vi "clear_multi_turn.vi"() -> ()   [LabVIEW 2016]
uses:
  dxl_x86_c.lvlib/dxl_x86_c.lvlib
panel:
  out "?":string
  in  "?":bool
  out "value : PRO (knob)\npresent position 2":i32(knob)
  out "value : PRO (knob)\npresent position":i32(knob) scale=150000.0..-150000.0
  in  "?":bool
  out "?":string
  in  "MAX_POSITION_VALUE":u32=1048575
  out "EXT_POSITION_\nCONTROL_MODE":dbl=4.0
  out "ADDR_\nOPERATING_MODE":u16
  in  "?":bool
  out "dynamixel_comm_result":string
  out "dynamixel_error":string
  in  "device_name":string="COM1"
  in  "ADDR_\nPRESENT_POSITION":u16=611
  in  "ADDR_\nGOAL_POSITION":u16=596
  in  "ADDR_\nTORQUE_ENABLE":u16=562
  out "protocol_version":dbl=2.0
  in  "?":bool
  out "port_num":i32
  in  "dynamixel_id":u8=1
  in  "baud_rate":i32=57600
  # "/*******************************************************************************\n* Copyright (c) 2016, ROBOTIS CO., LTD.\n* All rights reserved.\n*\n* Redistribution and use in source and binary forms, with or without\n* modification, are permitted provided that the following conditions are met:\n*\n* * Redistributions of source code must retain the above copyright notice, this\n*   list of conditions and the following disclaimer.\n*\n* * Redistributions in binary form must reproduce the above copyright notice,\n*   this list of conditions and the following disclaimer in the documentation\n*   and/or other materials provided with the distribution.\n*\n* * Neither the name of ROBOTIS nor the names of its\n*   contributors may be used to endorse or promote products derived from\n*   this software without specific prior written permission.\n*\n* THIS SOFTWARE IS PROVIDED BY THE COPYRIGHT HOLDERS AND CONTRIBUTORS \"AS IS\"\n* AND ANY EXPRESS OR IMPLIED WARRANTIES, INCLUDING, BUT NOT LIMITED TO, THE\n* IMPLIED WARRANTIES OF MERCHANTABILITY AND FITNESS FOR A PARTICULAR PURPOSE ARE\n* DISCLAIMED. IN NO EVENT SHALL THE COPYRIGHT HOLDER OR CONTRIBUTORS BE LIABLE\n* FOR ANY DIRECT, INDIRECT, INCIDENTAL, SPECIAL, EXEMPLARY, OR CONSEQUENTIAL\n* DAMAGES (INCLUDING, BUT NOT LIMITED TO, PROCUREMENT OF SUBSTITUTE GOODS OR\n* SERVICES; LOSS OF USE, DATA, OR PROFITS; OR BUSINESS INTERRUPTION) HOWEVER\n* CAUSED AND ON ANY THEORY OF LIABILITY, WHETHER IN CONTRACT, STRICT LIABILITY,\n* OR TORT (INCLUDING NEGLIGENCE OR OTHERWISE) ARISING IN ANY WAY OUT OF THE USE\n* OF THIS SOFTWARE, EVEN IF ADVISED OF THE POSSIBILITY OF SUCH DAMAGE.\n*******************************************************************************/\n\n/* Author: Ki Jong Gil (Gilbert) */"
  # "Available Dynamixel model on this example : All models using Protocol 2.0\nThis example is designed for using a Dynamixel X Series, and an USB2DYNAMIXEL.\nTo use another Dynamixel model, see their details in E-Manual(support.robotis.com) \nBe sure that Dynamixel X properties are already set as %% ID : 1 / Baudnum : 1 (Baudrate : 57600)\n\n1. Run example by click above \"Run\" button (below \"Edit\" menu).\n2. Click \"Start\" then you may see the Dynamixel and \"knob\" rotating\n3. When you want to clear turn, press \"Clear\" button.\n4. To contiue the turn, press \"Run\" button.\n3. To finish the example, press \"Stop\", \"Run\" and \"terminate\" button."
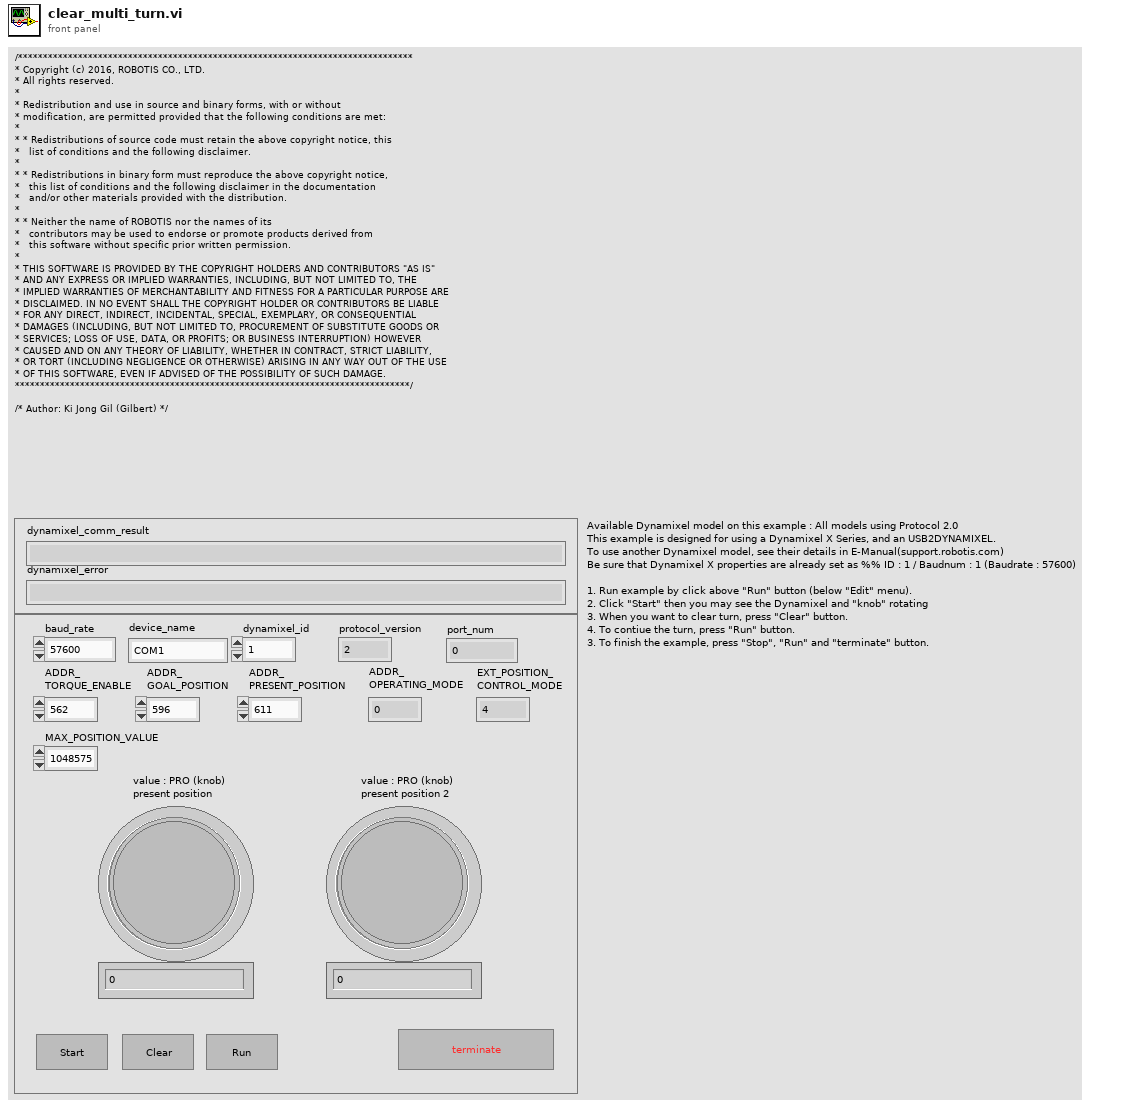
[diagram p1: front panel]
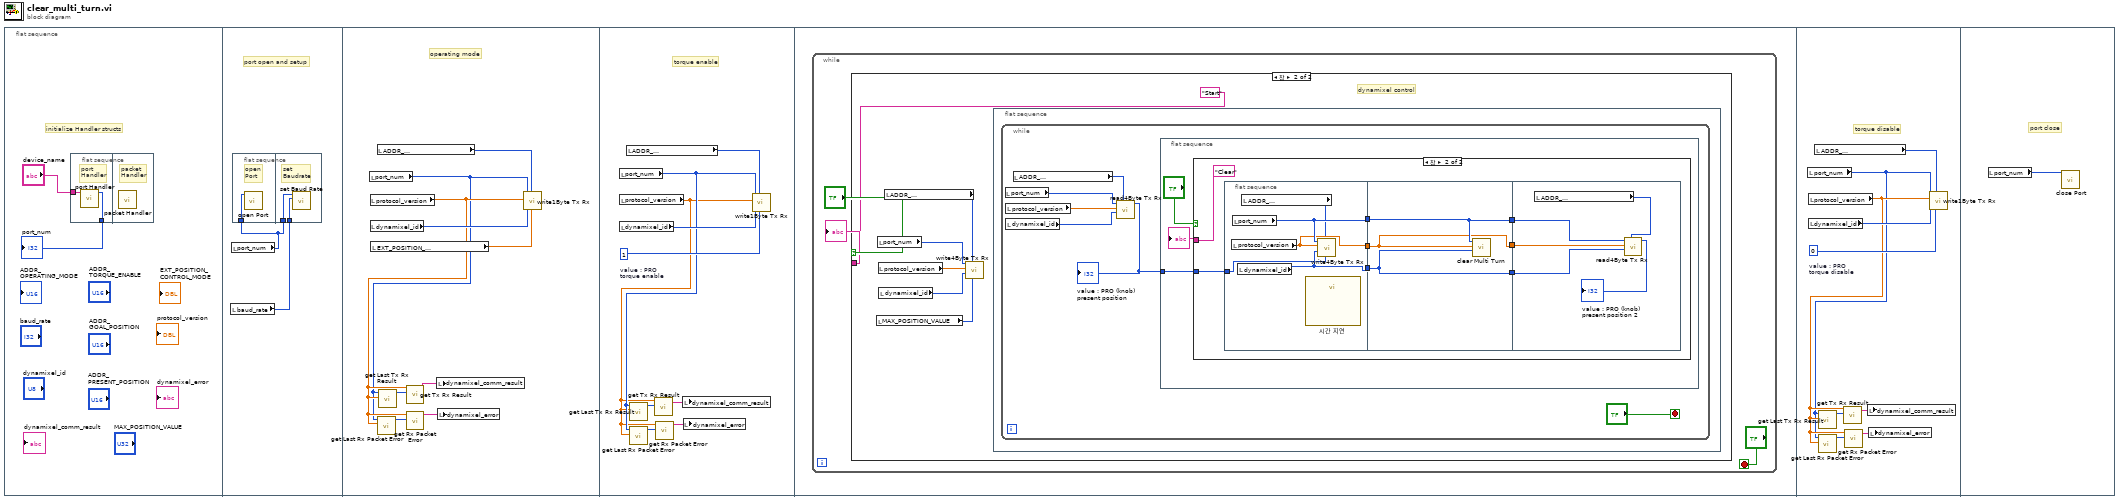
[diagram p0: block diagram]
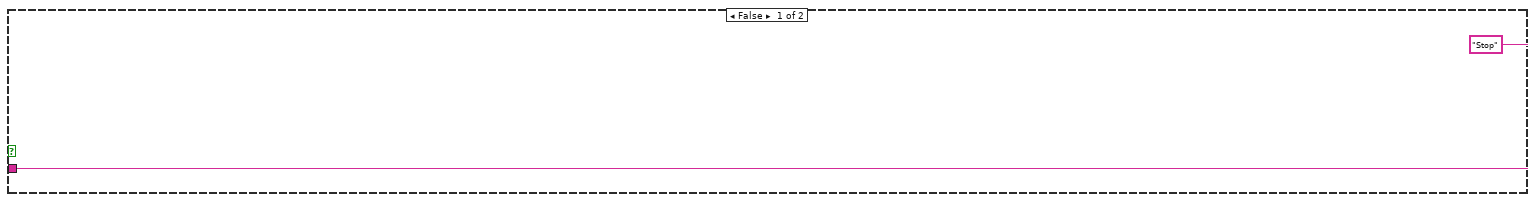
[diagram p2: hidden frame]
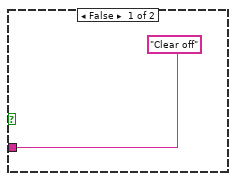
[diagram p3: hidden frame]
diagram:
  n1 = flat-sequence {
    frame #0 {
      # "initialize Handler structs"
      n2 = flat-sequence {
        tunnel: [w4] -> w2
        tunnel: "device_name" -> [w3]
        frame #0 {
          # "port\nHandler"
          n3 = call "port Handler.vi"("port_name"=w3) -> ("function return"=w4:i32)  [unwired: 10 in]
        }
        frame #1 {
          # "packet\nHandler"
          n4 = call "packet Handler.vi"() -> ()  [unwired: 12 in]
        }
      }
      "port_num" <- w2
    }
    frame #1 {
      # "port open and setup"
      n5 = local read "baud_rate"() -> (w5:i32)
      n6 = local read "port_num"() -> (w6:i32)
      n7 = flat-sequence {
        tunnel: w6 -> [w7]
        tunnel: w6 -> [w9]
        tunnel: w5 -> [w8]
        frame #0 {
          # "open\nPort"
          n8 = call "open Port.vi"("port_num"=w7) -> ()  [unwired: 10 in, 1 out]
        }
        frame #1 {
          # "set\nBaudrate"
          n9 = call "set Baud Rate.vi"("baudrate"=w8, "port_num"=w9) -> ()  [unwired: 9 in, 1 out]
        }
      }
    }
    frame #2 {
      # "operating mode"
      n10 = local read "port_num"() -> (w12:i32)
      n11 = local read "protocol_version"() -> (w13:dbl)
      n12 = local read "dynamixel_id"() -> (w18:u8)
      n13 = local read "EXT_POSITION_\nCONTROL_MODE"() -> (w16:dbl)
      n14 = local read "ADDR_\nOPERATING_MODE"() -> (w17:u16)
      n15 = call "get Last Rx Packet Error.vi"("protocol_version"=w13, "port_num"=w12) -> ("function return"=w14:u8)  [unwired: 9 in]
      n16 = call "get Last Tx Rx Result.vi"("protocol_version"=w13, "port_num"=w12) -> ("function return"=w15:i32)  [unwired: 9 in]
      n17 = call "get Tx Rx Result.vi"("result"=w15, "protocol_version"=w13) -> ("function return"=w10:string)  [unwired: 9 in]
      n18 = call "get Rx Packet Error.vi"("error"=w14, "protocol_version"=w13) -> ("function return"=w11:string)  [unwired: 9 in]
      n19 = local write "dynamixel_comm_result"(w10) -> ()
      n20 = local write "dynamixel_error"(w11) -> ()
      n21 = call "write1Byte Tx Rx.vi"("data"=w16, "address"=w17, "id"=w18, "protocol_version"=w13, "port_num"=w12) -> ()  [unwired: 7 in]
    }
    frame #3 {
      w27 = 1  # value : PRO torque enable
      # "torque enable"
      n22 = local read "port_num"() -> (w22:i32)
      n23 = local read "protocol_version"() -> (w21:dbl)
      n24 = local read "dynamixel_id"() -> (w26:u8)
      n25 = local read "ADDR_\nTORQUE_ENABLE"() -> (w25:u16)
      n26 = call "get Last Tx Rx Result.vi"("protocol_version"=w21, "port_num"=w22) -> ("function return"=w24:i32)  [unwired: 9 in]
      n27 = call "get Last Rx Packet Error.vi"("protocol_version"=w21, "port_num"=w22) -> ("function return"=w23:u8)  [unwired: 9 in]
      n28 = call "get Tx Rx Result.vi"("result"=w24, "protocol_version"=w21) -> ("function return"=w19:string)  [unwired: 9 in]
      n29 = call "get Rx Packet Error.vi"("error"=w23, "protocol_version"=w21) -> ("function return"=w20:string)  [unwired: 9 in]
      n30 = local write "dynamixel_comm_result"(w19) -> ()
      n31 = local write "dynamixel_error"(w20) -> ()
      n32 = call "write1Byte Tx Rx.vi"("data"=w27, "address"=w25, "id"=w26, "protocol_version"=w21, "port_num"=w22) -> ()  [unwired: 7 in]
    }
    frame #4 {
      n33 = while {
        stop <- "?" stop-if-true
        n34 = case shown="참" "?" {
          tunnel: ["Stop" "Start"] -> w29
          frame False {
          }
          frame True {
            # "dynamixel control"
            n35 = local read "MAX_POSITION_VALUE"() -> (w32:u32)
            n36 = local read "port_num"() -> (w33:i32)
            n37 = local read "protocol_version"() -> (w35:dbl)
            n38 = local read "dynamixel_id"() -> (w34:u8)
            n39 = local read "ADDR_\nGOAL_POSITION"() -> (w36:u16)
            n40 = call "write4Byte Tx Rx.vi"("data"=w32, "address"=w36, "id"=w34, "protocol_version"=w35, "port_num"=w33) -> ()  [unwired: 7 in]
            n41 = flat-sequence {
              frame #0 {
                n42 = while {
                  stop <- "?" stop-if-true
                  n43 = local read "port_num"() -> (w43:i32)
                  n44 = local read "protocol_version"() -> (w41:dbl)
                  n45 = local read "dynamixel_id"() -> (w42:u8)
                  n46 = local read "ADDR_\nPRESENT_POSITION"() -> (w40:u16)
                  n47 = call "read4Byte Tx Rx.vi"("address"=w40, "id"=w42, "protocol_version"=w41, "port_num"=w43) -> ("function return"=w39:u32)  [unwired: 7 in]
                  "value : PRO (knob)\npresent position" <- w39
                  n48 = flat-sequence {
                    tunnel: w39 -> [w44]
                    frame #0 {
                      n49 = case shown="참" "?" {
                        tunnel: ["Clear off" "Clear"] -> w46
                        tunnel: w44 -> [_ w48]
                        frame False {
                        }
                        frame True {
                          n50 = flat-sequence {
                            tunnel: [w60] -> w51
                            tunnel: [w59] -> w50
                            tunnel: [w58] -> w49
                            tunnel: w48 -> [w56]
                            tunnel: [w62] -> w54
                            tunnel: [w63] -> w53
                            tunnel: [w61] -> w52
                            tunnel: w51 -> [w63]
                            tunnel: w50 -> [w62]
                            tunnel: w49 -> [w61]
                            tunnel: w54 -> [w66]
                            tunnel: w53 -> [w65]
                            tunnel: w52 -> [w64]
                            frame #0 {
                              n51 = local read "protocol_version"() -> (w59:dbl)
                              n52 = local read "port_num"() -> (w60:i32)
                              n53 = local read "dynamixel_id"() -> (w58:u8)
                              n54 = local read "ADDR_\nGOAL_POSITION"() -> (w57:u16)
                              n55 = call "시간 지연"() -> ()  [unwired: 11 in, 1 out]
                              n56 = call "write4Byte Tx Rx.vi"("data"=w56, "address"=w57, "id"=w58, "protocol_version"=w59, "port_num"=w60) -> ()  [unwired: 7 in]
                            }
                            frame #1 {
                              n57 = call "clear Multi Turn.vi"("id"=w61, "protocol_version"=w62, "port_num"=w63) -> ()  [unwired: 9 in]
                            }
                            frame #2 {
                              n58 = local read "ADDR_\nPRESENT_POSITION"() -> (w68:u16)
                              n59 = call "read4Byte Tx Rx.vi"("address"=w68, "id"=w64, "protocol_version"=w66, "port_num"=w65) -> ("function return"=→"value : PRO (knob)\npresent position 2":u32)  [unwired: 7 in]
                            }
                          }
                        }
                      }
                      "?" <- w46
                    }
                  }
                }
              }
            }
          }
        }
        "?" <- w29
      }
    }
    frame #5 {
      w76 = 0  # value : PRO torque disable
      # "torque disable"
      n60 = local read "port_num"() -> (w71:i32)
      n61 = local read "protocol_version"() -> (w72:dbl)
      n62 = local read "dynamixel_id"() -> (w77:u8)
      n63 = local read "ADDR_\nTORQUE_ENABLE"() -> (w75:u16)
      n64 = call "get Last Tx Rx Result.vi"("protocol_version"=w72, "port_num"=w71) -> ("function return"=w73:i32)  [unwired: 9 in]
      n65 = call "get Last Rx Packet Error.vi"("protocol_version"=w72, "port_num"=w71) -> ("function return"=w74:u8)  [unwired: 9 in]
      n66 = call "get Tx Rx Result.vi"("result"=w73, "protocol_version"=w72) -> ("function return"=w70:string)  [unwired: 9 in]
      n67 = call "get Rx Packet Error.vi"("error"=w74, "protocol_version"=w72) -> ("function return"=w69:string)  [unwired: 9 in]
      n68 = local write "dynamixel_comm_result"(w70) -> ()
      n69 = local write "dynamixel_error"(w69) -> ()
      n70 = call "write1Byte Tx Rx.vi"("data"=w76, "address"=w75, "id"=w77, "protocol_version"=w72, "port_num"=w71) -> ()  [unwired: 7 in]
    }
    frame #6 {
      # "port close"
      n71 = local read "port_num"() -> (w78:i32)
      n72 = call "close Port.vi"("port_num"=w78) -> ()  [unwired: 11 in]
    }
  }
